vi "Build Arrays with For Loops.vi"() -> ()   [LabVIEW 2019]
panel:
  out "number: 0 to 1":dbl
  out "Array":dbl[](array[numeric])
  out "Random Number":dbl
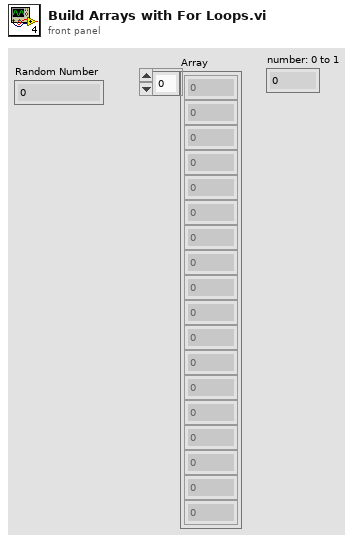
[diagram p1: front panel]
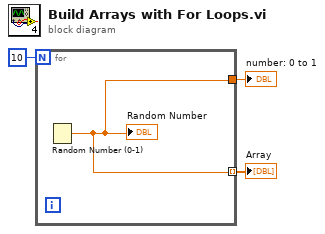
[diagram p0: block diagram]
diagram:
  n1 = for {
    N: 10 -> [_]
    tunnel: [w4] -> w2 mode=indexing
    tunnel: [w4] -> w1
    n2 = Random Number (0-1)() -> (number: 0 to 1=w4:dbl)
    "Random Number" <- w4
  }
  "Array" <- w2
  "number: 0 to 1" <- w1
